vi "draw_2d.vi"(10 "ID":dbl) -> (2 "appended array":cluster{dbl[], dbl[]}[](array[cluster]))   [LabVIEW 2011]
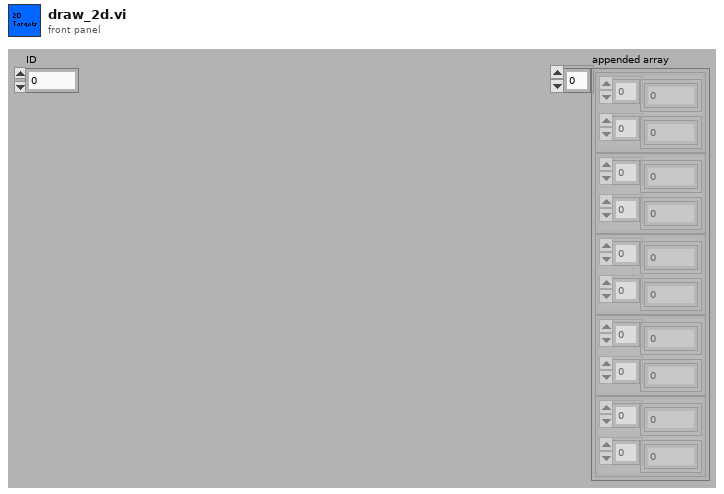
[diagram p1: front panel]
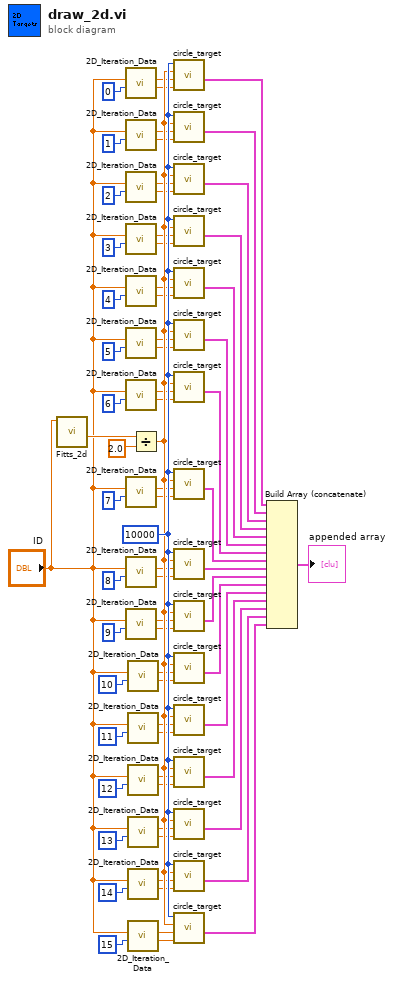
[diagram p0: block diagram]
diagram:
  w70 = 10000 ("Pixels")
  n1 = call "Fitts_2d.vi"("ID"="ID") -> ("W"=w69:dbl)  [unwired: 9 in, 1 out]
  n2 = call "2D_Iteration_Data.vi"("Iteration"=0, "ID"="ID") -> ("y0"=w64:dbl, "x0"=w65:dbl)  [unwired: 8 in]
  n3 = call "2D_Iteration_Data.vi"("Iteration"=1, "ID"="ID") -> ("y0"=w62:dbl, "x0"=w63:dbl)  [unwired: 8 in]
  n4 = call "2D_Iteration_Data.vi"("Iteration"=2, "ID"="ID") -> ("y0"=w60:dbl, "x0"=w61:dbl)  [unwired: 8 in]
  n5 = call "2D_Iteration_Data.vi"("Iteration"=3, "ID"="ID") -> ("y0"=w58:dbl, "x0"=w59:dbl)  [unwired: 8 in]
  n6 = call "2D_Iteration_Data.vi"("Iteration"=4, "ID"="ID") -> ("y0"=w56:dbl, "x0"=w57:dbl)  [unwired: 8 in]
  n7 = call "2D_Iteration_Data.vi"("Iteration"=5, "ID"="ID") -> ("y0"=w54:dbl, "x0"=w55:dbl)  [unwired: 8 in]
  n8 = call "2D_Iteration_Data.vi"("Iteration"=6, "ID"="ID") -> ("y0"=w52:dbl, "x0"=w53:dbl)  [unwired: 8 in]
  n9 = call "2D_Iteration_Data.vi"("Iteration"=7, "ID"="ID") -> ("y0"=w50:dbl, "x0"=w51:dbl)  [unwired: 8 in]
  n10 = call "2D_Iteration_Data.vi"("Iteration"=8, "ID"="ID") -> ("y0"=w48:dbl, "x0"=w49:dbl)  [unwired: 8 in]
  n11 = call "2D_Iteration_Data.vi"("Iteration"=9, "ID"="ID") -> ("y0"=w46:dbl, "x0"=w47:dbl)  [unwired: 8 in]
  n12 = call "2D_Iteration_Data.vi"("Iteration"=10, "ID"="ID") -> ("y0"=w44:dbl, "x0"=w45:dbl)  [unwired: 8 in]
  n13 = call "2D_Iteration_Data.vi"("Iteration"=11, "ID"="ID") -> ("y0"=w42:dbl, "x0"=w43:dbl)  [unwired: 8 in]
  n14 = call "2D_Iteration_Data.vi"("Iteration"=12, "ID"="ID") -> ("y0"=w40:dbl, "x0"=w41:dbl)  [unwired: 8 in]
  n15 = call "2D_Iteration_Data.vi"("Iteration"=13, "ID"="ID") -> ("y0"=w38:dbl, "x0"=w39:dbl)  [unwired: 8 in]
  n16 = call "2D_Iteration_Data.vi"("Iteration"=14, "ID"="ID") -> ("y0"=w36:dbl, "x0"=w37:dbl)  [unwired: 8 in]
  n17 = call "2D_Iteration_Data.vi"("Iteration"=15, "ID"="ID") -> ("y0"=w34:dbl, "x0"=w35:dbl)  [unwired: 8 in]
  n18 = Divide(x=w69, y=2.0) -> (x/y=w67:dbl)
  n19 = call "circle_target.vi"("y0"=w64, "x0"=w65, "Radius"=w67, "Pixels"=w70) -> ("Target plots"=w16:cluster{dbl[], dbl[]}[])  [unwired: 7 in]
  n20 = call "circle_target.vi"("y0"=w62, "x0"=w63, "Radius"=w67, "Pixels"=w70) -> ("Target plots"=w15:cluster{dbl[], dbl[]}[])  [unwired: 7 in]
  n21 = call "circle_target.vi"("y0"=w60, "x0"=w61, "Radius"=w67, "Pixels"=w70) -> ("Target plots"=w14:cluster{dbl[], dbl[]}[])  [unwired: 7 in]
  n22 = call "circle_target.vi"("y0"=w58, "x0"=w59, "Radius"=w67, "Pixels"=w70) -> ("Target plots"=w13:cluster{dbl[], dbl[]}[])  [unwired: 7 in]
  n23 = call "circle_target.vi"("y0"=w56, "x0"=w57, "Radius"=w67, "Pixels"=w70) -> ("Target plots"=w12:cluster{dbl[], dbl[]}[])  [unwired: 7 in]
  n24 = call "circle_target.vi"("y0"=w54, "x0"=w55, "Radius"=w67, "Pixels"=w70) -> ("Target plots"=w11:cluster{dbl[], dbl[]}[])  [unwired: 7 in]
  n25 = call "circle_target.vi"("y0"=w52, "x0"=w53, "Radius"=w67, "Pixels"=w70) -> ("Target plots"=w10:cluster{dbl[], dbl[]}[])  [unwired: 7 in]
  n26 = call "circle_target.vi"("y0"=w50, "x0"=w51, "Radius"=w67, "Pixels"=w70) -> ("Target plots"=w9:cluster{dbl[], dbl[]}[])  [unwired: 7 in]
  n27 = call "circle_target.vi"("y0"=w48, "x0"=w49, "Radius"=w67, "Pixels"=w70) -> ("Target plots"=w8:cluster{dbl[], dbl[]}[])  [unwired: 7 in]
  n28 = call "circle_target.vi"("y0"=w46, "x0"=w47, "Radius"=w67, "Pixels"=w70) -> ("Target plots"=w7:cluster{dbl[], dbl[]}[])  [unwired: 7 in]
  n29 = call "circle_target.vi"("y0"=w44, "x0"=w45, "Radius"=w67, "Pixels"=w70) -> ("Target plots"=w6:cluster{dbl[], dbl[]}[])  [unwired: 7 in]
  n30 = call "circle_target.vi"("y0"=w42, "x0"=w43, "Radius"=w67, "Pixels"=w70) -> ("Target plots"=w5:cluster{dbl[], dbl[]}[])  [unwired: 7 in]
  n31 = call "circle_target.vi"("y0"=w40, "x0"=w41, "Radius"=w67, "Pixels"=w70) -> ("Target plots"=w4:cluster{dbl[], dbl[]}[])  [unwired: 7 in]
  n32 = call "circle_target.vi"("y0"=w38, "x0"=w39, "Radius"=w67, "Pixels"=w70) -> ("Target plots"=w3:cluster{dbl[], dbl[]}[])  [unwired: 7 in]
  n33 = call "circle_target.vi"("y0"=w36, "x0"=w37, "Radius"=w67, "Pixels"=w70) -> ("Target plots"=w2:cluster{dbl[], dbl[]}[])  [unwired: 7 in]
  n34 = call "circle_target.vi"("y0"=w34, "x0"=w35, "Radius"=w67, "Pixels"=w70) -> ("Target plots"=w1:cluster{dbl[], dbl[]}[])  [unwired: 7 in]
  n35 = Build Array (concatenate)(w16, w15, w14, w13, w12, w11, w10, w9, w8, w7, w6, w5, w4, w3, w2, w1) -> (→"appended array":cluster{dbl[], dbl[]}[])
